vi "MagX Filter Info.vi"(8 "error in":errorcluster, 10 "Search":string, 11 "Data in":T1[](array[typedef])) -> (0 "error out":errorcluster, 3 "Data out":T1[](array[typedef]))   [LabVIEW 2024]
uses:
  Experiment info.ctl
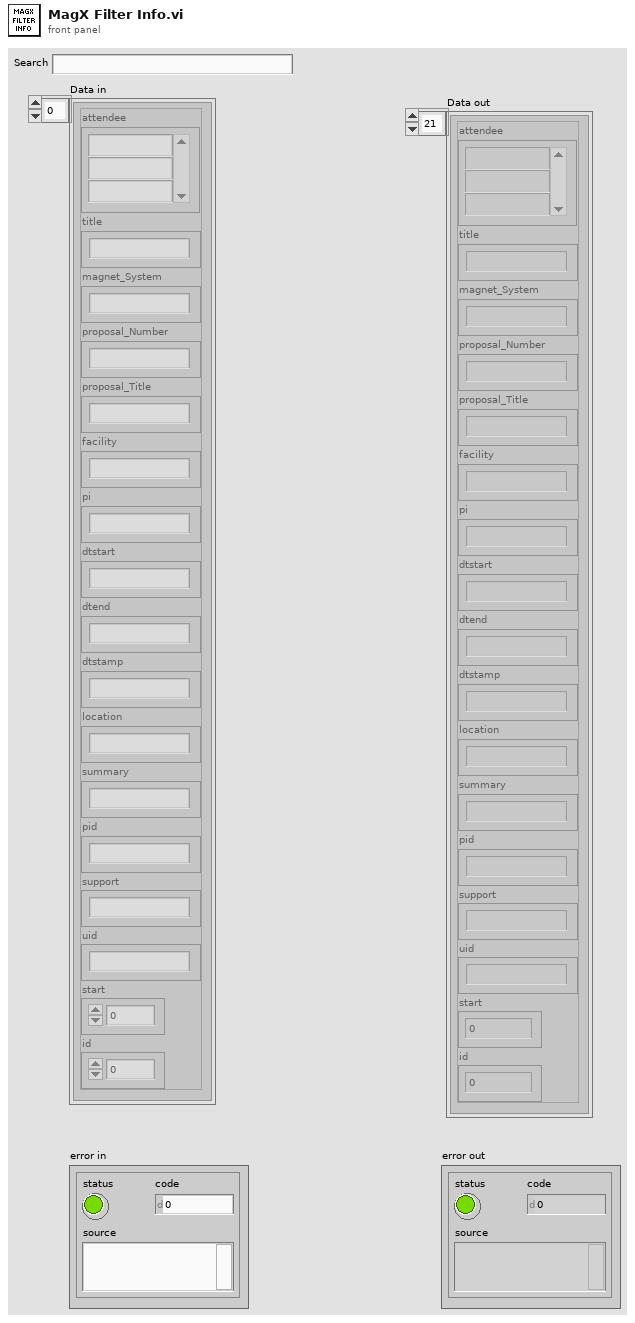
[diagram p1: front panel]
types:
  T1 = typedef "Experiment info.ctl" = cluster{"attendee":string[], "title":string, "magnet_System":string, "proposal_Number":string, "proposal_Title":string, "facility":string, "pi":string, "dtstart":string, "dtend":string, "dtstamp":string, "location":string, "summary":string, "pid":string, "support":string, "uid":string, "start":u64, "id":u64}
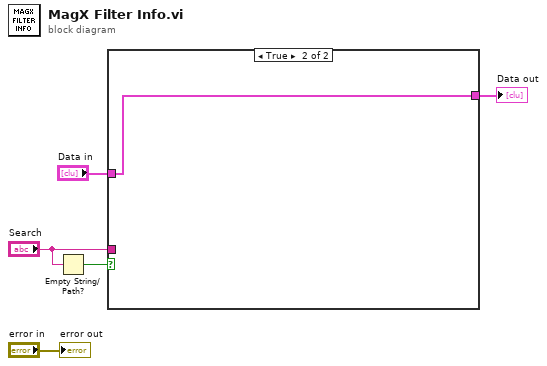
[diagram p0: block diagram]
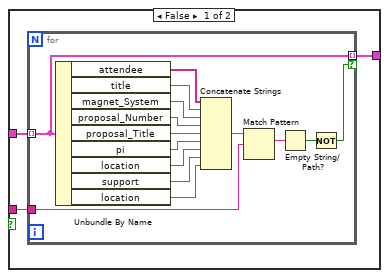
[diagram p2: hidden frame]
diagram:
  n1 = Empty String/Path?(string/path="Search") -> (empty?=w1:bool)
  n2 = case shown="True" w1 {
    tunnel: "Data in" -> [w8 w24]
    tunnel: [w7 w24] -> w4
    tunnel: "Search" -> [w6 _]
    frame False {
      n3 = for {
        tunnel: w8 -> [w23] mode=indexing
        tunnel: [w23] -> w7 mode=indexing if=w9
        tunnel: w6 -> [w22]
        n4 = Unbundle By Name(w23) -> ("attendee"=w21:string[], "title"=w20:string, "magnet_System"=w19:string, "proposal_Number"=w18:string, "proposal_Title"=w17:string, "pi"=w16:string, "location"=w15:string, "support"=w14:string, "location"=w13:string)
        n5 = Concatenate Strings(w21, w20, w19, w18, w17, w16, w15, w14, w13) -> (w12:string)
        n6 = Match Pattern(string=w12, regular expression=w22) -> (match substring=w11:string)  [unwired: 1 in, 3 out]
        n7 = Empty String/Path?(string/path=w11) -> (empty?=w10:bool)
        n8 = Not(x=w10) -> (.not. x?=w9:bool)
      }
    }
    frame True {
    }
  }
  "Data out" <- w4
  "error out" <- "error in"
